vi "Enable Sync Output.vi"(8 "error in (no error)":errorcluster, 10 "Enable Sync Output (T: Enable)":bool=TRUE, 11 "VISA resource name":refnum<visa-resource-name>) -> (0 "error out":errorcluster, 3 "VISA resource name out":refnum<visa-resource-name>)   [LabVIEW 2010, in "AWG.lvlib" / "Agilent 3352X Series.lvlib"]
doc: "Disables or enables the output of front-panel Sync connector. \nYou can configure the Sync output using Configure Sync Output.VI located in Configure/Output Configration"
uses:
  Agilent 3352X Series.lvlib
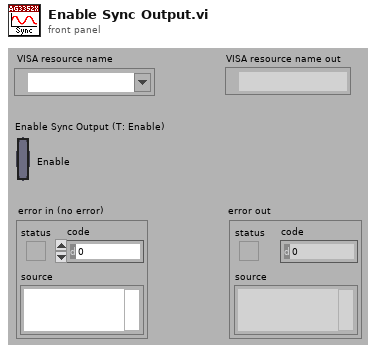
[diagram p1: front panel]
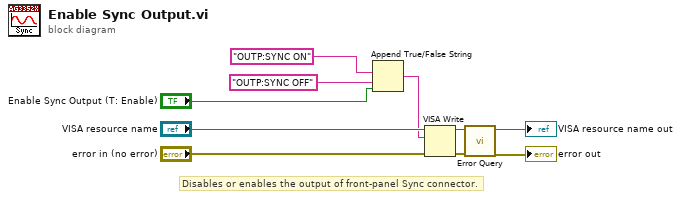
[diagram p0: block diagram]
diagram:
  # "Disables or enables the output of front-panel Sync connector."
  n1 = Append True/False String(1:"Enable Sync Output (T: Enable)", 2:"OUTP:SYNC OFF", 3:"OUTP:SYNC ON") -> (0:w1:string)  [unwired: 1 out]
  n2 = VISA Write(VISA resource name="VISA resource name", write buffer=w1, error in (no error)="error in (no error)") -> (VISA resource name out=w5:refnum<visa-resource-name>, error out=w4:errorcluster)  [unwired: 1 out]
  n3 = call "Error Query.vi"("error in (no error)"=w4, "VISA resource name"=w5) -> ("error out"=→"error out":errorcluster, "VISA resource name out"=→"VISA resource name out":refnum<visa-resource-name>)  [unwired: 8 out]
